vi "Tiempo.vi"() -> (0 "Dt":dbl)   [LabVIEW 2011]
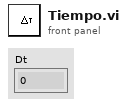
[diagram p1: front panel]
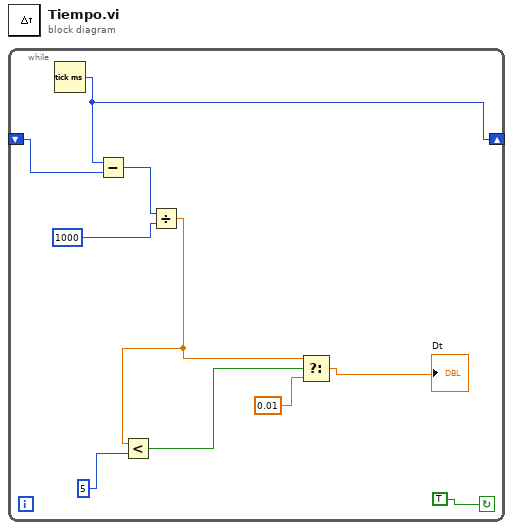
[diagram p0: block diagram]
diagram:
  n1 = while {
    shift-right: [w8] -> _
    shift-left: _ -> [w9]
    stop <- TRUE continue-if-true
    n2 = Tick Count (ms)() -> (millisecond timer value=w8:u32)
    n3 = Subtract(x=w8, y=w9) -> (x-y=w7:u32)
    n4 = Divide(x=w7, y=1000) -> (x/y=w1:dbl)
    n5 = Less?(x=w1, y=5) -> (x < y?=w5:bool)
    n6 = Select(t=w1, s=w5, f=0.01) -> (s? t:f=→"Dt":dbl)
  }
